vi "Create Top Level.vi"(9 "Alias":string, 10 "Actor":refnum<class "LVCAM.lvclass">) -> ()   [LabVIEW 2021, in "LVCAM.lvlib" / "Actor.lvclass"]
uses:
  Actor.lvclass
  Msg/Msg.lvclass
  LVCAM/LVCAM.lvclass
  C:/PPLs/LabVIEW-Composed-Actor-Model-LVCAM/LabVIEW-Composed-Actor-Model-LVCAM/LVCAM/LVCAM/LVCAM/LVCAM.lvclass
  C:/PPLs/LabVIEW-Composed-Actor-Model-LVCAM/LabVIEW-Composed-Actor-Model-LVCAM/LVCAM/Msgs/LVCAM Create Nest/LVCAM Create Nest/LVCAM Create Nest.lvclass
  C:/PPLs/LabVIEW-Composed-Actor-Model-LVCAM/LabVIEW-Composed-Actor-Model-LVCAM/LVCAM/Msgs/LVCAM Destroy Self/LVCAM Destroy Self/LVCAM Destroy Self.lvclass
  C:/PPLs/LabVIEW-Composed-Actor-Model-LVCAM/LabVIEW-Composed-Actor-Model-LVCAM/LVCAM/Msgs/LVCAM Nest Destroyed/LVCAM Nest Destroyed/LVCAM Nest Destroyed.lvclass
  C:/PPLs/LabVIEW-Composed-Actor-Model-LVCAM/LabVIEW-Composed-Actor-Model-LVCAM/LVCAM/LVCAM/LVCAM Create/LVCAM Create.lvclass
  C:/PPLs/LabVIEW-Composed-Actor-Model-LVCAM/LabVIEW-Composed-Actor-Model-LVCAM/LVCAM/LVCAM/LVCAM Destroy/LVCAM Destroy.lvclass
  C:/PPLs/LabVIEW-Composed-Actor-Model-LVCAM/LabVIEW-Composed-Actor-Model-LVCAM/LVCAM/LVCAM/LVCAM Receive/LVCAM Receive.lvclass
  C:/PPLs/LabVIEW-Composed-Actor-Model-LVCAM/LabVIEW-Composed-Actor-Model-LVCAM/LVCAM/LVCAM/Actor/Actor.lvclass
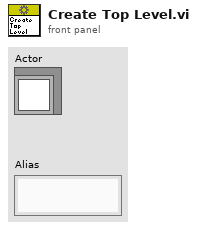
[diagram p1: front panel]
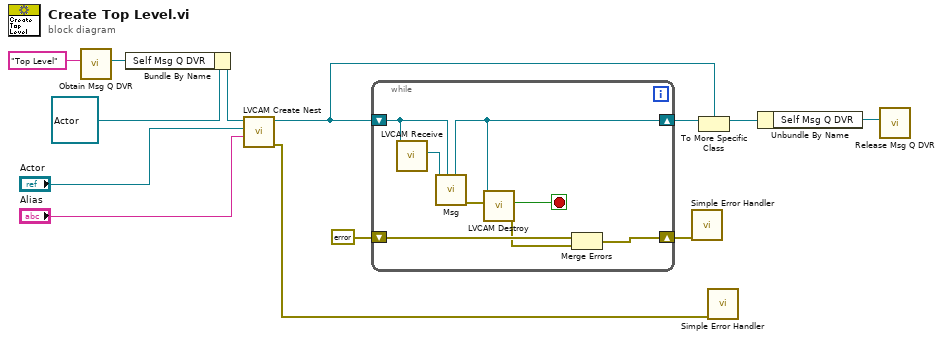
[diagram p0: block diagram]
diagram:
  n1 = call "Obtain Msg Q DVR.vi"("Msg Q DVR Alias"="Top Level") -> ("Msg Q DVR"=w10:refnum<data-value>)  [unwired: 9 in, 1 out]
  n2 = Bundle By Name(cluster=refnum<class "Actor.lvclass"> refnum ("Self Actor in"), "Self Msg Q DVR"=w10) -> (w11:refnum<class "Actor.lvclass">)
  n3 = call-dynamic "LVCAM Create Nest.vi"("Nest Alias"="Alias", "Nest Actor"="Actor", "Actor in"=w11) -> ("error out"=w9:errorcluster, "Actor out"=w1:refnum<class "Actor.lvclass">)  [unwired: 7 in]
  n4 = while {
    shift-right: [w17] -> w7
    shift-left: w1 -> [w19]
    shift-right: [w20] -> w8
    shift-left: errorcluster {"status"=FALSE, "code"=0, "source"=""} ("error out") -> [w18]
    stop <- w14 stop-if-true
    n5 = call-dynamic "LVCAM Receive.vi"("LVCAM Receive in"=w19) -> ("Msg"=w21:refnum<class "Msg.lvclass">)  [unwired: 9 in, 1 out]
    n6 = call-dynamic "Msg.vi"("ABD in"=w19, "Msg in"=w21) -> ("error out"=w16:errorcluster, "ABD out"=w17:refnum<class "LVCAM.lvclass">)  [unwired: 8 in]
    n7 = call-dynamic "LVCAM Destroy.vi"("Error"=w16, "LVCAM Destroy in"=w17) -> ("error out"=w15:errorcluster, "Destroyed?"=w14:bool)  [unwired: 7 in, 1 out]
    n8 = Merge Errors(w18, w15) -> (w20:errorcluster)
  }
  n9 = call <vilib>:"Simple Error Handler.vi"("error in (no error)"=w8) -> ()  [unwired: 4 in, 5 out]
  n10 = To More Specific Class(target class=w1, reference=w7) -> (specific class reference=w2:refnum<class "Actor.lvclass">)  [unwired: 1 in, 1 out]
  n11 = call <vilib>:"Simple Error Handler.vi"("error in (no error)"=w9) -> ()  [unwired: 4 in, 5 out]
  n12 = Unbundle By Name(w2) -> ("Self Msg Q DVR"=w6:refnum<data-value>)
  n13 = call "Release Msg Q DVR.vi"("Msg Q DVR"=w6) -> ()  [unwired: 10 in, 1 out]
